vi "PLC DATA READ.vi"() -> ()   [LabVIEW 2021]
uses:
  <vilib>/Hampel Software Engineering/S7NetCom/Source/PDU Size --ring.ctl
  <vilib>/Hampel Software Engineering/S7NetCom/Source/Controls/S7_Memory_Area.ctl
  <vilib>/Hampel Software Engineering/S7NetCom/Source/API/Read Data - Boolean (Scalar).vi
  <vilib>/Hampel Software Engineering/S7NetCom/Source/API/Read Data - Real (Scalar).vi
  <vilib>/Hampel Software Engineering/S7NetCom/Source/API/Write Data - Real (Scalar).vi
  <vilib>/Hampel Software Engineering/S7NetCom/Source/S7NetCom.lvclass
panel:
  out "Real Value":sgl
  in  "Value":sgl
  out "Boolean Value":bool
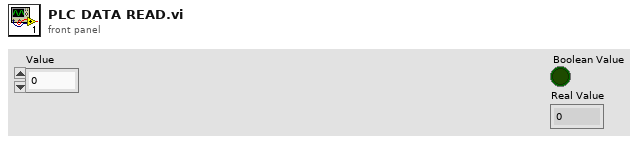
[diagram p1: front panel]
types:
  T1 = typedef "S7NetCom.lvlib/S7NetCom.lvclass/S7_Memory_Area.ctl" = enum8{"P Area", "I Area", "O Area", "M Area", "DB Area", "Counter", "Timer"}
  T2 = typedef "S7NetCom.lvlib/S7NetCom.lvclass/PDU Size --ring.ctl" = u16
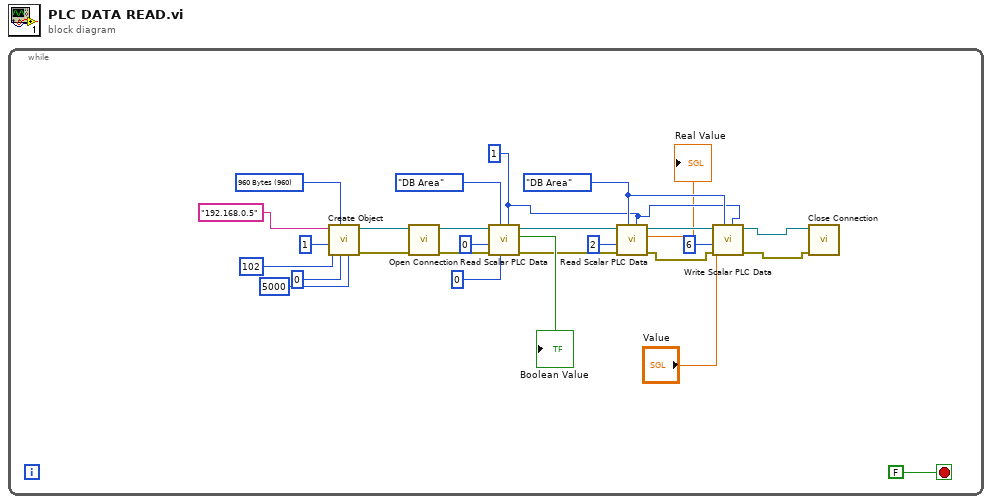
[diagram p0: block diagram]
diagram:
  n1 = while {
    stop <- FALSE stop-if-true
    w6 = S7_Memory_Area."DB Area" ("Memory Area")
    w5 = u16 1 ("Data Block #")
    w23 = T2 960 items=["240 Bytes"=240, "480 Bytes"=480, "960 Bytes"=960] ("PDU Size")
    n2 = call <vilib>:"Create Object.vi"("Timeout"=5000, "Rack"=u8 0, "PDU Size"=w23, "Slot"=u8 1, "Port"=u16 102, "IP Address"="192.168.0.5") -> ("error out"=w27:errorcluster, "S7NetCom out"=w26:refnum<class "S7NetCom.lvclass">)  [unwired: 4 in]
    n3 = call <vilib>:"Open Connection.vi"("error in"=w27, "S7NetCom in"=w26) -> ("error out"=w18:errorcluster, "S7NetCom out"=w19:refnum<class "S7NetCom.lvclass">)  [unwired: 8 in]
    n4 = call-poly <vilib>:"Read Scalar PLC Data.vi"("Data Block #"=w5, "Bit Offset"=u8 0, "Memory Area"=S7_Memory_Area."DB Area", "error in (no error)"=w18, "Start Address"=u32 0, "S7 in"=w19) -> ("error out"=w11:errorcluster, "Boolean Value"=→"Boolean Value":bool, "S7 out"=w12:refnum<class "S7NetCom.lvclass">)  [unwired: 3 in]
    n5 = call-poly <vilib>:"Read Scalar PLC Data.vi"("Data Block #"=w5, "Memory Area"=w6, "error in (no error)"=w11, "Start Address"=u32 2, "S7 in"=w12) -> ("error out"=w9:errorcluster, "Real Value"=→"Real Value":sgl, "S7 out"=w10:refnum<class "S7NetCom.lvclass">)  [unwired: 4 in]
    n6 = call-poly <vilib>:"Write Scalar PLC Data.vi"("Data Block #"=w5, "Memory Area"=w6, "error in (no error)"=w9, "Start Address"=u32 6, "Value"="Value", "S7 in"=w10) -> ("error out"=w7:errorcluster, "S7 out"=w8:refnum<class "S7NetCom.lvclass">)  [unwired: 4 in]
    n7 = call <vilib>:"Close Connection.vi"("error in (no error)"=w7, "S7NetCom in"=w8) -> ()  [unwired: 8 in, 2 out]
  }
